vi "myRIO_BRig_RT__Case_Exp_State_Cue1__v3.vi"(7 "I_lick":bool, 8 "input_arrTrig":bool[](array[boolean]), 10 "input_state":T1, 11 "input_dataCurrent":u16[](array[numeric])) -> (0 "output_l1_laserOn":bool, 1 "output_l1_laserEvent":bool, 2 "output_state":T1, 3 "output_dataCurrent":u16[](array[numeric]), 4 "output_l2_laserEvent":bool, 5 "output_CueLed_Event":bool, 6 "output_l2_laserOn":bool)   [LabVIEW 2014]
uses:
  myRIO_BRig_RT__Case_Exp_stateList.ctl
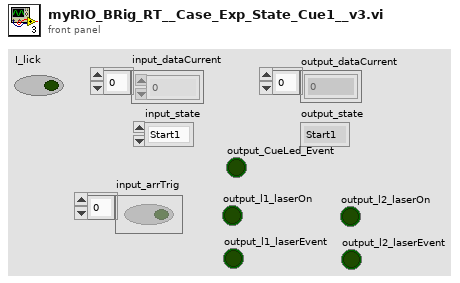
[diagram p1: front panel]
types:
  T1 = typedef "myRIO_BRig_RT__Case_Exp_stateList.ctl" = enum16{"Start1", "Start2", "Start3", "saveSettings1", "saveSettings2", "saveSettings3", "saveSettings4", "saveSettings_LC_ENL_l1", "saveSettings_LC_ENL_l2", "saveSettings_LC_Cue_l1", "saveSettings_LC_Cue_l2", "saveSettings6_LC_l1_Other", "SaveSettings6_LC_l2_Other", "setSettings_Audio", "setSettings_Laser", "initBlock_pre", "initBlock", "initBlock2", "initBlock_post", "initTrial_pre", "initTrial", "initTrial2", "initTrial3", "initTrial4", "initTrial_LC_ENL1", "initTrial_LC_Cue1", "initTrial_LC_Cue1_2", "initTrial_LC_Sel", "initTrial_post", "ENL1_pre", "ENL1", "ENL1_post", "ENL1Penalty_pre", "ENL1Penalty", "ENL2_pre", "ENL2", "ENL2Penalty_pre", "ENL2Penalty", "Cue1_pre", "Cue1", "Cue1_post", "Cue1Penalty_pre", "Cue1Penalty", "Cue2_pre", "Cue2", "Cue2Penalty_pre", "Cue2Penalty", "Selection_pre", "Selection", "Select_post", "SelectReward_pre", "SelectReward", "SelectRewardPost_pre", "SelectRewardPost", "SelectWrong_pre", "SelectWrong", "SelectWrong_post", "SelectTimeout_pre", "SelectTimeout", "SelectTimeout_post", "endTrial_pre", "endTrial1", "endTrial2", "endTrial3", "endTrial_post", "endBlock_pre", "endBlock", "endBlock_post", "endExp", "commConnect", "commUpload_pre", "commUpload_dataBlock", "commUpload_dataCurrent", "commUpload_dataExp", "commUpload_dataLC", "commUpload_dataTrial", "commUpload_post", "saveData_pre", "saveData_dataBlock", "saveData_dataCurrent", "saveData_dataExp", "saveData_dataLC", "saveData_dataTrial", "saveData_post", "empty_endBlock1", "empty_endBlock2", "empty_endTrial1", "empty_endTrial2", "empty_endTrial3", "empty_endTrial4", "empty_endTrial5", "dummyState", "dummyState_endBlock"}
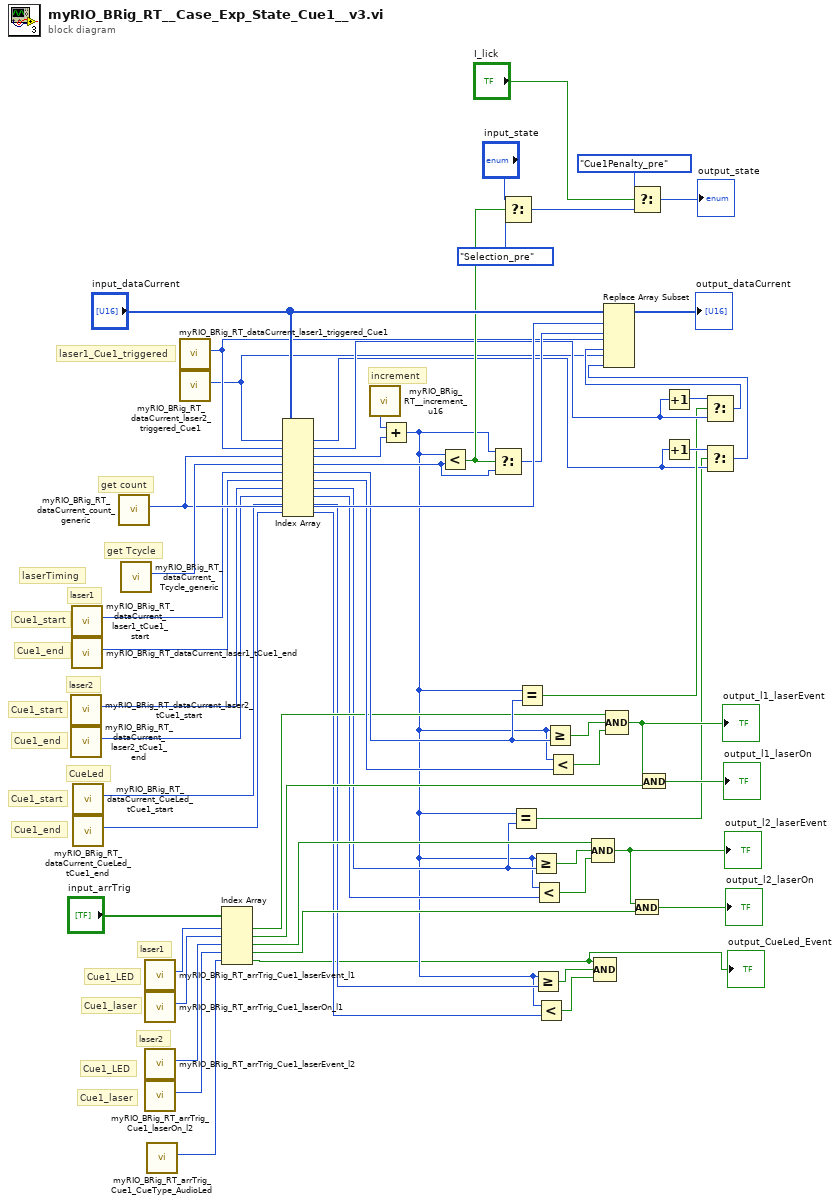
[diagram p0: block diagram]
diagram:
  # "Cue1_end"
  # "Cue1_start"
  # "CueLed"
  # "Cue1_LED"
  # "Cue1_laser"
  # "Cue1_LED"
  # "Cue1_laser"
  # "laser2"
  # "laser1"
  # "Cue1_end"
  # "Cue1_start"
  # "laser2"
  # "laser1"
  # "Cue1_end"
  # "Cue1_start"
  # "laser1_Cue1_triggered"
  # "laserTiming"
  # "increment"
  # "get Tcycle"
  # "get count"
  n1 = call "myRIO_BRig_RT_dataCurrent_laser2_tCue1_start.vi"() -> ("output_laser2_tCue1_start"=w32:i32)  [unwired: 11 in]
  n2 = call "myRIO_BRig_RT_dataCurrent_laser2_tCue1_end.vi"() -> ("output_laser2_tCue1_end"=w31:i32)  [unwired: 11 in]
  n3 = call "myRIO_BRig_RT_dataCurrent_laser1_tCue1_start.vi"() -> ("output_laser1_tCue1_start"=w34:i32)  [unwired: 11 in]
  n4 = call "myRIO_BRig_RT_dataCurrent_laser1_tCue1_end.vi"() -> ("output_laser1_tCue1_end"=w33:i32)  [unwired: 11 in]
  n5 = call "myRIO_BRig_RT_dataCurrent_CueLed_tCue1_start.vi"() -> ("output_CueLed_tCue1_start"=w16:i32)  [unwired: 11 in]
  n6 = call "myRIO_BRig_RT_dataCurrent_CueLed_tCue1_end.vi"() -> ("output_CueLed_tCue1_end"=w15:i32)  [unwired: 11 in]
  n7 = call "myRIO_BRig_RT_dataCurrent_count_generic.vi"() -> ("output_count_generic"=w56:i32)  [unwired: 11 in]
  n8 = call "myRIO_BRig_RT_dataCurrent_Tcycle_generic.vi"() -> ("output_Tcycle_generic"=w57:i32)  [unwired: 11 in]
  n9 = call "myRIO_BRig_RT_arrTrig_Cue1_laserEvent_l1.vi"() -> ("output_arrTrig_Cue1_laserEvent_l1"=w29:i32)  [unwired: 11 in]
  n10 = call "myRIO_BRig_RT_arrTrig_Cue1_laserOn_l1.vi"() -> ("output_arrTrig_Cue1_laserOn_l1"=w28:i32)  [unwired: 11 in]
  n11 = call "myRIO_BRig_RT_arrTrig_Cue1_laserEvent_l2.vi"() -> ("output_arrTrig_Cue1_laserEvent_l2"=w27:i32)  [unwired: 11 in]
  n12 = call "myRIO_BRig_RT_arrTrig_Cue1_laserOn_l2.vi"() -> ("output_arrTrig_Cue1_laserOn_l2"=w26:i32)  [unwired: 11 in]
  n13 = call "myRIO_BRig_RT_arrTrig_Cue1_CueType_AudioLed.vi"() -> ("output_arrTrig_Cue1_CueType_AudioLed"=w10:i32)  [unwired: 11 in]
  n14 = call "myRIO_BRig_RT_dataCurrent_laser1_triggered_Cue1.vi"() -> ("output_laser1_triggered_Cue1"=w40:i32)  [unwired: 11 in]
  n15 = call "myRIO_BRig_RT_dataCurrent_laser2_triggered_Cue1.vi"() -> ("output_laser2_triggered_Cue1"=w9:i32)  [unwired: 11 in]
  n16 = Index Array(array="input_arrTrig", index #1=w29, index #2=w28, index #3=w27, index #4=w26, index #5=w10) -> (element #1=w24:bool, element #2=w25:bool, element #3=w23:bool, element #4=w22:bool, element #5=w1:bool)
  "output_CueLed_Event" <- w1
  n17 = Index Array(array="input_dataCurrent", index #1=w9, index #2=w40, index #3=w56, index #4=w57, index #5=w34, index #6=w33, index #7=w32, index #8=w31, index #9=w16, index #10=w15) -> (element #1=w6:u16, element #2=w38:u16, element #3=w36:u16, element #4=w55:u16, element #5=w35:u16, element #6=w42:u16, element #7=w4:u16, element #8=w21:u16, element #9=w14:u16, element #10=w13:u16)
  n18 = call "myRIO_BRig_RT__increment_u16.vi"() -> ("output_increment__u16"=w50:u16)  [unwired: 11 in]
  n19 = Add(x=w50, y=w36) -> (x+y=w3:u16)
  n20 = Less?(x=w3, y=w55) -> (x < y?=w52:bool)
  n21 = Select(t=w3, s=w52, f=w55) -> (s? t:f=w54:u16)
  n22 = Select(t="input_state", s=w52, f=myRIO_BRig_RT__Case_Exp_stateList."Selection_pre" ("Enum")) -> (s? t:f=w51:T1)
  n23 = Equal?(x=w3, y=w4) -> (x = y?=w2:bool)
  n24 = Equal?(x=w3, y=w35) -> (x = y?=w7:bool)
  n25 = Greater Or Equal?(x=w3, y=w4) -> (x >= y?=w20:bool)
  n26 = Greater Or Equal?(x=w3, y=w14) -> (x >= y?=w12:bool)
  n27 = Less?(x=w3, y=w21) -> (x < y?=w19:bool)
  n28 = Less?(x=w3, y=w13) -> (x < y?=w11:bool)
  n29 = Greater Or Equal?(x=w3, y=w35) -> (x >= y?=w48:bool)
  n30 = Less?(x=w3, y=w42) -> (x < y?=w49:bool)
  n31 = Compound Arithmetic op=AND(w23, w20, w19) -> (w18:bool)
  "output_l2_laserEvent" <- w18
  n32 = Compound Arithmetic op=AND(w1, w12, w11) -> ()  [unwired: 1 out]
  n33 = Compound Arithmetic op=AND(w24, w48, w49) -> (w37:bool)
  "output_l1_laserEvent" <- w37
  n34 = Select(t=myRIO_BRig_RT__Case_Exp_stateList."Cue1Penalty_pre" ("Enum"), s="I_lick", f=w51) -> (s? t:f=→"output_state":T1)
  n35 = And(x=w18, y=w22) -> (x .and. y?=→"output_l2_laserOn":bool)
  n36 = And(x=w37, y=w25) -> (x .and. y?=→"output_l1_laserOn":bool)
  n37 = Increment(x=w38) -> (x+1=w39:u16)
  n38 = Increment(x=w6) -> (x+1=w8:u16)
  n39 = Select(t=w39, s=w7, f=w38) -> (s? t:f=w41:u16)
  n40 = Select(t=w8, s=w2, f=w6) -> (s? t:f=w5:u16)
  n41 = Replace Array Subset(array="input_dataCurrent", new element #1=w54, index #1=w56, new element #2=w41, index #2=w40, new element #3=w5, index #3=w9) -> (→"output_dataCurrent":u16[])
